vi "svfa_Window Frequency Response (first derivative, double).vi"(1 "N (window length)":i32, 2 "window":T1(ring), 3 "f(normalized)":dbl format="%.5e") -> (0 "H'(f)":dbl format="%.5e")   [LabVIEW 2017]
uses:
  <vilib>/addons/_NISVFA/_Spectrum Processing/subVIs/svfa_Rect Window Frequency Response.vi
  <vilib>/addons/_NISVFA/_Spectrum Processing/subVIs/svfa_Cosine Window Coefficients.vi
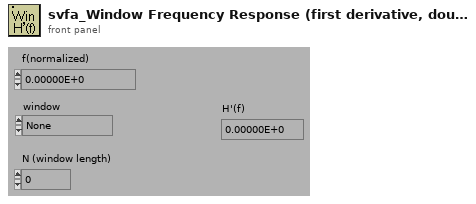
[diagram p1: front panel]
types:
  T1 = enum16{"None ", "Hanning", "Hamming", "Blackman-Harris", "Exact Blackman", "Blackman", "Flat Top", "4 Term B-Harris ", "7 Term B-Harris", "Low Sidelobe"}
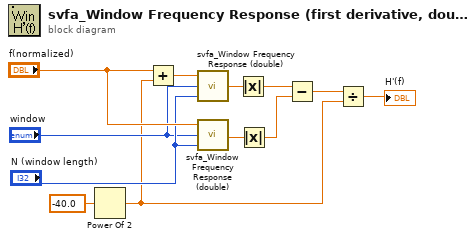
[diagram p0: block diagram]
diagram:
  n1 = Power Of 2(x=-40.0) -> (2^x=w2:dbl)
  n2 = Add(x="f(normalized)", y=w2) -> (x+y=w12:dbl)
  n3 = call <vilib>:"svfa_Window Frequency Response (double).vi"("N (window length)"="N (window length)", "window"="window", "f(normalized)"=w12) -> ("H(f)"=w7:cdb)
  n4 = call <vilib>:"svfa_Window Frequency Response (double).vi"("N (window length)"="N (window length)", "window"="window", "f(normalized)"="f(normalized)") -> ("H(f)"=w6:cdb)
  n5 = Absolute Value(x=w7) -> (abs(x)=w5:dbl)
  n6 = Absolute Value(x=w6) -> (abs(x)=w4:dbl)
  n7 = Subtract(x=w5, y=w4) -> (x-y=w3:dbl)
  n8 = Divide(x=w3, y=w2) -> (x/y=→"H'(f)":dbl)
